vi "RT Host - normalised time profile.vi"(7 "Which speed profile?":T1, 8 "Error In":errorcluster, 11 "X Input (normalised 0-1)":dbl) -> (0 "Error Out":errorcluster, 2 "Profile Mean":dbl format="%0.2f", 3 "Y output (normalised 0-1)":dbl)   [LabVIEW 2017]
doc: "This subVI provides a Y-value according to a defined x-input by interpolating a senables multiple normailsed profiles to be created and followed according to."
uses:
  Controls/hCAAR - speed profile.ctl
  <vilib>/Analysis/baseanly.llb/Mean (DBL).vi
  <vilib>/Analysis/1siggen.llb/Ramp Pattern by Samples.vi
  <vilib>/Analysis/NI_AALPro.lvlib
  <vilib>/Analysis/NI_AALBase.lvlib
panel:
  out "Time V Distance Profile":cluster{dbl[], "Interpolant":dbl[]}(graph)={[0.0, 0.010101010101010102, 0.020202020202020204, 0.030303030303030304, 0.04040404040404041, 0.050505050505050504, 0.06060606060606061, 0.0707070707070707, 0.08080808080808081, 0.09090909090909091, 0.10101010101010101, 0.1111111111111111, 0.12121212121212122, 0.13131313131313133, 0.1414141414141414, 0.15151515151515152, 0.16161616161616163, 0.1717171717171717, 0.18181818181818182, 0.1919191919191919, 0.20202020202020202, 0.21212121212121213, 0.2222222222222222, 0.23232323232323232, 0.24242424242424243, 0.25252525252525254, 0.26262626262626265, 0.2727272727272727, 0.2828282828282828, 0.29292929292929293, 0.30303030303030304, 0.31313131313131315, 0.32323232323232326, 0.3333333333333333, 0.3434343434343434, 0.35353535353535354, 0.36363636363636365, 0.37373737373737376, 0.3838383838383838, 0.3939393939393939, 0.40404040404040403, 0.41414141414141414, 0.42424242424242425, 0.43434343434343436, 0.4444444444444444, 0.45454545454545453, 0.46464646464646464, 0.47474747474747475, 0.48484848484848486, 0.494949494949495, 0.5050505050505051, 0.5151515151515151, 0.5252525252525253, 0.5353535353535354, 0.5454545454545454, 0.5555555555555556, 0.5656565656565656, 0.5757575757575758, 0.5858585858585859, 0.5959595959595959, 0.6060606060606061, 0.6161616161616161, 0.6262626262626263, 0.6363636363636364, 0.6464646464646465, 0.6565656565656566, 0.6666666666666666, 0.6767676767676768, 0.6868686868686869, 0.696969696969697, 0.7070707070707071, 0.7171717171717171, 0.7272727272727273, 0.7373737373737373, 0.7474747474747475, 0.7575757575757576, 0.7676767676767676, 0.7777777777777778, 0.7878787878787878, 0.797979797979798, 0.8080808080808081, 0.8181818181818182, 0.8282828282828283, 0.8383838383838383, 0.8484848484848485, 0.8585858585858586, 0.8686868686868687, 0.8787878787878788, 0.8888888888888888, 0.898989898989899, 0.9090909090909091, 0.9191919191919192, 0.9292929292929293, 0.9393939393939394, 0.9494949494949495, 0.9595959595959596, 0.9696969696969697, 0.9797979797979798, 0.98989898989899, 1.0], "Interpolant"=[0.0, 0.03141075907812829, 0.06279051952931337, 0.09410831331851431, 0.12533323356430423, 0.15643446504023087, 0.1873813145857246, 0.21814324139654254, 0.24868988716485477, 0.2789911060392292, 0.3090169943749474, 0.33873792024529137, 0.3681245526846779, 0.3971478906347806, 0.4257792915650726, 0.4539904997395468, 0.4817536741017152, 0.5090414157503713, 0.5358267949789965, 0.5620833778521306, 0.587785252292473, 0.6129070536529765, 0.6374239897486896, 0.6613118653236518, 0.6845471059286886, 0.7071067811865475, 0.7289686274214114, 0.7501110696304595, 0.7705132427757891, 0.7901550123756903, 0.8090169943749473, 0.8270805742745617, 0.844327925502015, 0.8607420270039435, 0.8763066800438635, 0.8910065241883678, 0.9048270524660195, 0.917754625683981, 0.9297764858882513, 0.9408807689542253, 0.9510565162951535, 0.960293685676943, 0.9685831611286311, 0.9759167619387473, 0.9822872507286886, 0.9876883405951377, 0.9921147013144778, 0.99556196460308, 0.9980267284282716, 0.9995065603657316, 1.0, 0.9995065603657316, 0.9980267284282716, 0.9955619646030801, 0.9921147013144779, 0.9876883405951379, 0.9822872507286887, 0.9759167619387475, 0.9685831611286312, 0.9602936856769432, 0.9510565162951536, 0.9408807689542256, 0.9297764858882515, 0.9177546256839813, 0.9048270524660196, 0.891006524188368, 0.8763066800438637, 0.8607420270039438, 0.8443279255020152, 0.8270805742745619, 0.8090169943749476, 0.7901550123756905, 0.7705132427757894, 0.7501110696304597, 0.7289686274214117, 0.7071067811865477, 0.6845471059286888, 0.661311865323652, 0.6374239897486899, 0.6129070536529767, 0.5877852522924732, 0.5620833778521308, 0.5358267949789968, 0.5090414157503715, 0.48175367410171543, 0.453990499739547, 0.4257792915650728, 0.39714789063478084, 0.36812455268467814, 0.3387379202452916, 0.3090169943749476, 0.27899110603922944, 0.248689887164855, 0.21814324139654273, 0.18738131458572485, 0.15643446504023106, 0.12533323356430448, 0.09410831331851452, 0.06279051952931362, 0.03141075907812849]}
  out "Speed V Time Profile":cluster{dbl[], "Interpolant":dbl[]}(graph)={[0.0, 0.010101010101010102, 0.020202020202020204, 0.030303030303030304, 0.04040404040404041, 0.050505050505050504, 0.06060606060606061, 0.0707070707070707, 0.08080808080808081, 0.09090909090909091, 0.10101010101010101, 0.1111111111111111, 0.12121212121212122, 0.13131313131313133, 0.1414141414141414, 0.15151515151515152, 0.16161616161616163, 0.1717171717171717, 0.18181818181818182, 0.1919191919191919, 0.20202020202020202, 0.21212121212121213, 0.2222222222222222, 0.23232323232323232, 0.24242424242424243, 0.25252525252525254, 0.26262626262626265, 0.2727272727272727, 0.2828282828282828, 0.29292929292929293, 0.30303030303030304, 0.31313131313131315, 0.32323232323232326, 0.3333333333333333, 0.3434343434343434, 0.35353535353535354, 0.36363636363636365, 0.37373737373737376, 0.3838383838383838, 0.3939393939393939, 0.40404040404040403, 0.41414141414141414, 0.42424242424242425, 0.43434343434343436, 0.4444444444444444, 0.45454545454545453, 0.46464646464646464, 0.47474747474747475, 0.48484848484848486, 0.494949494949495, 0.5050505050505051, 0.5151515151515151, 0.5252525252525253, 0.5353535353535354, 0.5454545454545454, 0.5555555555555556, 0.5656565656565656, 0.5757575757575758, 0.5858585858585859, 0.5959595959595959, 0.6060606060606061, 0.6161616161616161, 0.6262626262626263, 0.6363636363636364, 0.6464646464646465, 0.6565656565656566, 0.6666666666666666, 0.6767676767676768, 0.6868686868686869, 0.696969696969697, 0.7070707070707071, 0.7171717171717171, 0.7272727272727273, 0.7373737373737373, 0.7474747474747475, 0.7575757575757576, 0.7676767676767676, 0.7777777777777778, 0.7878787878787878, 0.797979797979798, 0.8080808080808081, 0.8181818181818182, 0.8282828282828283, 0.8383838383838383, 0.8484848484848485, 0.8585858585858586, 0.8686868686868687, 0.8787878787878788, 0.8888888888888888, 0.898989898989899, 0.9090909090909091, 0.9191919191919192, 0.9292929292929293, 0.9393939393939394, 0.9494949494949495, 0.9595959595959596, 0.9696969696969697, 0.9797979797979798, 0.98989898989899, 1.0], "Interpolant"=[0.0, 0.03141075907812829, 0.06279051952931337, 0.09410831331851431, 0.12533323356430423, 0.15643446504023087, 0.1873813145857246, 0.21814324139654254, 0.24868988716485477, 0.2789911060392292, 0.3090169943749474, 0.33873792024529137, 0.3681245526846779, 0.3971478906347806, 0.4257792915650726, 0.4539904997395468, 0.4817536741017152, 0.5090414157503713, 0.5358267949789965, 0.5620833778521306, 0.587785252292473, 0.6129070536529765, 0.6374239897486896, 0.6613118653236518, 0.6845471059286886, 0.7071067811865475, 0.7289686274214114, 0.7501110696304595, 0.7705132427757891, 0.7901550123756903, 0.8090169943749473, 0.8270805742745617, 0.844327925502015, 0.8607420270039435, 0.8763066800438635, 0.8910065241883678, 0.9048270524660195, 0.917754625683981, 0.9297764858882513, 0.9408807689542253, 0.9510565162951535, 0.960293685676943, 0.9685831611286311, 0.9759167619387473, 0.9822872507286886, 0.9876883405951377, 0.9921147013144778, 0.99556196460308, 0.9980267284282716, 0.9995065603657316, 1.0, 0.9995065603657316, 0.9980267284282716, 0.9955619646030801, 0.9921147013144779, 0.9876883405951379, 0.9822872507286887, 0.9759167619387475, 0.9685831611286312, 0.9602936856769432, 0.9510565162951536, 0.9408807689542256, 0.9297764858882515, 0.9177546256839813, 0.9048270524660196, 0.891006524188368, 0.8763066800438637, 0.8607420270039438, 0.8443279255020152, 0.8270805742745619, 0.8090169943749476, 0.7901550123756905, 0.7705132427757894, 0.7501110696304597, 0.7289686274214117, 0.7071067811865477, 0.6845471059286888, 0.661311865323652, 0.6374239897486899, 0.6129070536529767, 0.5877852522924732, 0.5620833778521308, 0.5358267949789968, 0.5090414157503715, 0.48175367410171543, 0.453990499739547, 0.4257792915650728, 0.39714789063478084, 0.36812455268467814, 0.3387379202452916, 0.3090169943749476, 0.27899110603922944, 0.248689887164855, 0.21814324139654273, 0.18738131458572485, 0.15643446504023106, 0.12533323356430448, 0.09410831331851452, 0.06279051952931362, 0.03141075907812849]}
  in  "User-Defined":cluster{"X":dbl, "Y":dbl}[](array[cluster])=[{"X"=0.0, "Y"=0.0}, {"X"=0.0600000000000001, "Y"=0.13000000000000006}, {"X"=0.10999999999999996, "Y"=0.2999999999999998}, {"X"=0.17999999999999988, "Y"=0.5299999999999998}, {"X"=0.33999999999999997, "Y"=0.8599999999999999}, {"X"=0.47, "Y"=0.98}, {"X"=0.61, "Y"=0.99}, {"X"=0.8, "Y"=0.8600000000000001}, {"X"=0.8800000000000001, "Y"=0.5800000000000001}, {"X"=0.9500000000000001, "Y"=0.19000000000000006}, {"X"=1.0, "Y"=0.0}] {"Y" step=0.01; "X" step=0.01}
  # "Outputs"
  # "Inputs"
  # "Local Data"
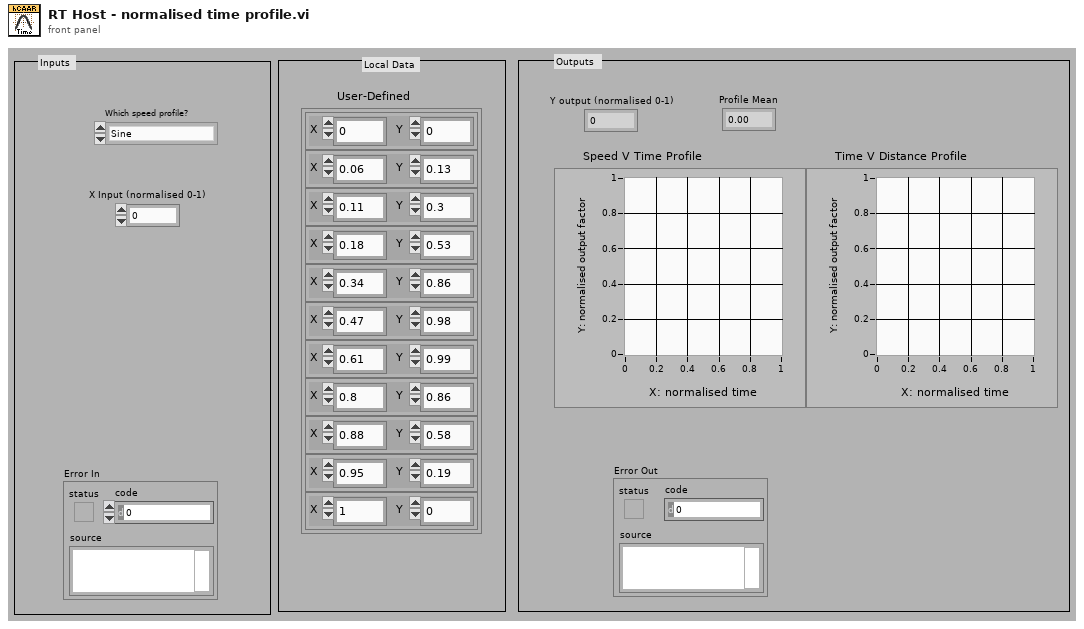
[diagram p1: front panel]
types:
  T1 = typedef "hCAAR - speed profile.ctl" = enum16{"Sine", "Sine With Initial Shunt", "Triangle", "Square", "Sawtooth", "Forward Skew", "User Defined"}
  T2 = enum16{"sine", "cosine", "triangle", "square", "sawtooth", "increasing ramp", "decreasing ramp"}
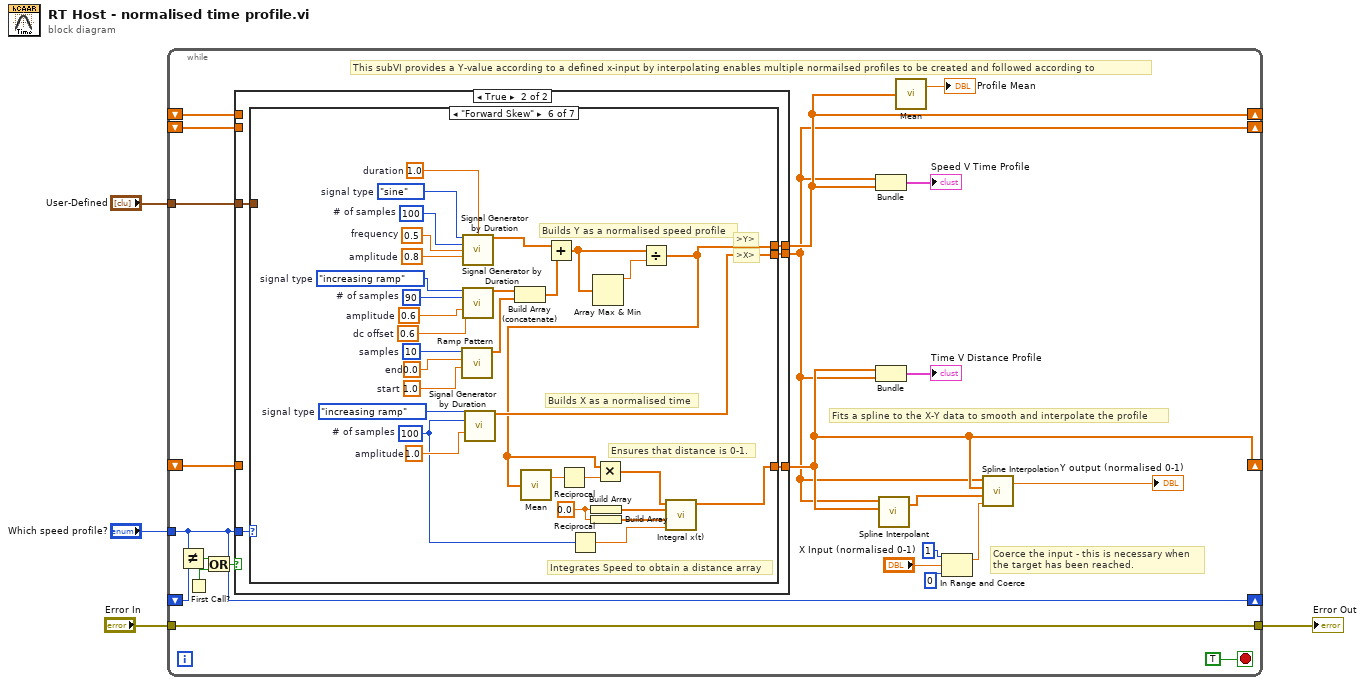
[diagram p0: block diagram]
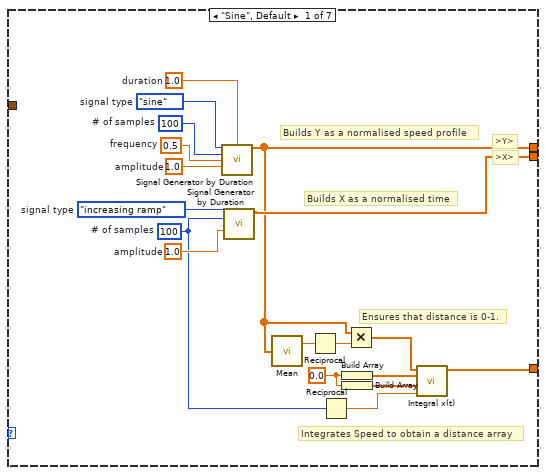
[diagram p3: hidden frame]
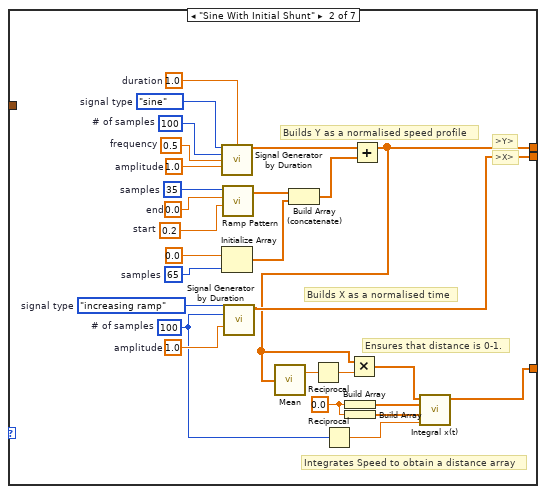
[diagram p4: hidden frame]
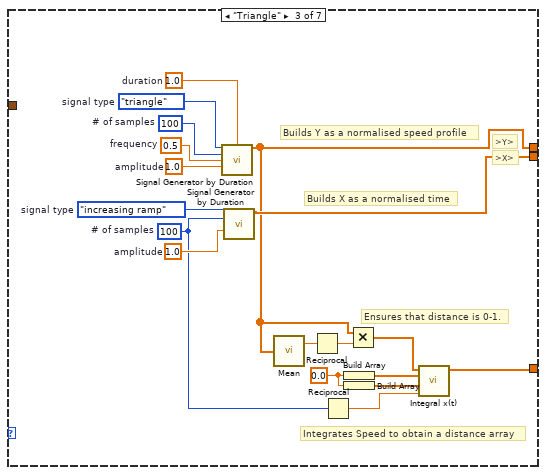
[diagram p5: hidden frame]
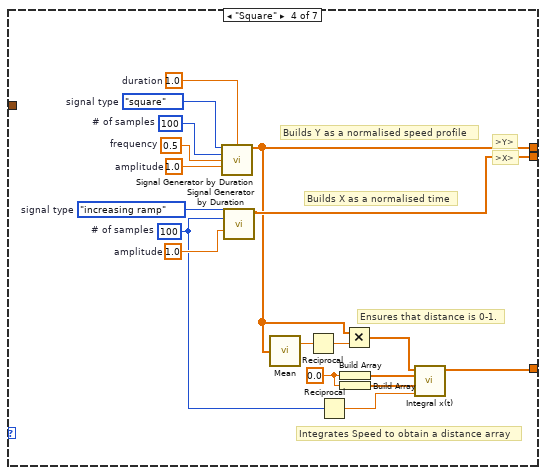
[diagram p6: hidden frame]
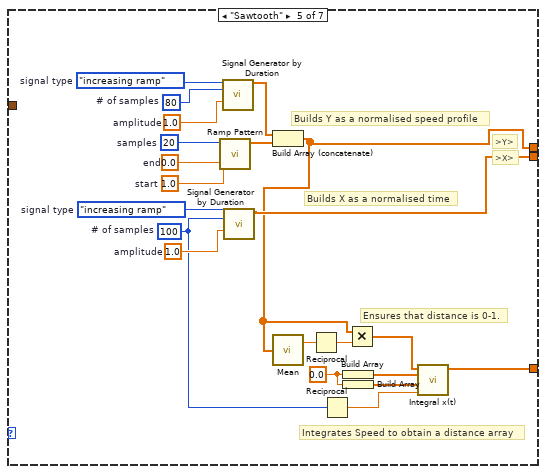
[diagram p7: hidden frame]
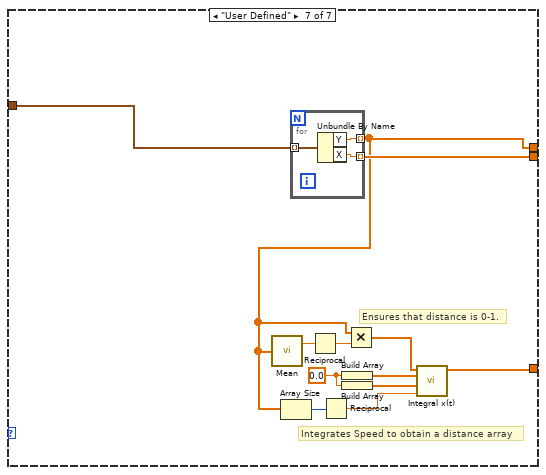
[diagram p8: hidden frame]
diagram:
  n1 = while {
    tunnel: "User-Defined" -> [w27]
    tunnel: "Which speed profile?" -> [w16]
    tunnel: [w20] -> w2
    tunnel: "Error In" -> [w20]
    shift-right: [w14] -> _
    shift-left: _ -> [w18]
    shift-right: [w6] -> _
    shift-left: _ -> [w17]
    shift-right: [w16] -> _
    shift-left: _ -> [w15]
    shift-right: [w7] -> _
    shift-left: _ -> [w9]
    stop <- TRUE stop-if-true
    # "This subVI provides a Y-value according to a defined x-input by interpolating enables multiple normailsed profiles to be created and followed according to"
    # "Fits a spline to the X-Y data to smooth and interpolate the profile"
    # "Coerce the input - this is necessary when\nthe target has been reached."
    n2 = Not Equal?(x=w16, y=w15) -> (x != y?=w12:bool)
    n3 = First Call?() -> (First Call?: T/F=w10:bool)
    n4 = Or(x=w12, y=w10) -> (x .or. y?=w11:bool)
    n5 = case shown="True" w11 {
      tunnel: w27 -> [_ w35]
      tunnel: w16 -> [_ w34]
      tunnel: [w29 w33] -> w6
      tunnel: [w30 w32] -> w14
      tunnel: w18 -> [w30 _]
      tunnel: w17 -> [w29 _]
      tunnel: [w28 w31] -> w7
      tunnel: w9 -> [w28 _]
      frame False {
        # "Saves CPU by only generating a new profile array when the profile type is changed"
      }
      frame True {
        n6 = case shown="\"Forward Skew\"" w34 {
          tunnel: [w46 w72 w91 w109 w135 w161 w180] -> w33
          tunnel: [w37 w55 w81 w100 w118 w139 w170] -> w32
          tunnel: w35 -> [_ _ _ _ _ _ w179]
          tunnel: [w38 w56 w86 w101 w119 w140 w171] -> w31
          frame "Sine", Default {
            w43 = 0.0
            w36 = 100  # # of samples
            w47 = 1.0  # amplitude
            w48 = T2."increasing ramp"  # signal type
            w49 = 1.0  # duration
            w50 = 100  # # of samples
            w51 = 0.5  # frequency
            w52 = 1.0  # amplitude
            w53 = T2."sine"  # signal type
            # "Ensures that distance is 0-1."
            # "Integrates Speed to obtain a distance array"
            # "Builds Y as a normalised speed profile"
            # "Builds X as a normalised time"
            # ">X>"
            # ">Y>"
            n7 = call <vilib>:"Signal Generator by Duration.vi"("signal type"=w53, "duration"=w49, "# of samples"=w50, "frequency"=w51, "amplitude"=w52) -> ("signal"=w37:dbl[])  [unwired: 7 in, 3 out]
            n8 = call <vilib>:"Signal Generator by Duration.vi"("signal type"=w48, "# of samples"=w36, "amplitude"=w47) -> ("signal"=w46:dbl[])  [unwired: 9 in, 3 out]
            n9 = call-poly <vilib>:"Mean.vi"("X"=w37) -> ("mean"=w41:dbl)  [unwired: 1 out]
            n10 = Reciprocal(x=w41) -> (1/x=w39:dbl)
            n11 = Reciprocal(x=w36) -> (1/x=w42:dbl)
            n12 = Build Array(w43) -> (w45:dbl[])
            n13 = Build Array(w43) -> (w44:dbl[])
            n14 = Multiply(x=w37, y=w39) -> (x*y=w40:dbl[])
            n15 = call <vilib>:"Integral x(t).vi"("dt"=w42, "Final Condition"=w44, "Initial Condition"=w45, "X"=w40) -> ("Integral X"=w38:dbl[])  [unwired: 6 in, 1 out]
          }
          frame "Sine With Initial Shunt" {
            w61 = 0.0
            w70 = 65  # samples
            w65 = 0.2  # start
            w67 = 0.0  # end
            w66 = 35  # samples
            w54 = 100  # # of samples
            w73 = 1.0  # amplitude
            w74 = T2."increasing ramp"  # signal type
            w76 = 1.0  # duration
            w77 = 100  # # of samples
            w78 = 0.5  # frequency
            w79 = 1.0  # amplitude
            w80 = T2."sine"  # signal type
            # "Ensures that distance is 0-1."
            # "Integrates Speed to obtain a distance array"
            # "Builds Y as a normalised speed profile"
            # "Builds X as a normalised time"
            # ">X>"
            # ">Y>"
            n16 = call <vilib>:"Signal Generator by Duration.vi"("signal type"=w80, "duration"=w76, "# of samples"=w77, "frequency"=w78, "amplitude"=w79) -> ("signal"=w75:dbl[])  [unwired: 7 in, 3 out]
            n17 = Initialize Array(0.0 ("element"), w70) -> (w71:dbl[])
            n18 = call-poly <vilib>:"Ramp Pattern.vi"("start"=w65, "end"=w67, "samples"=w66) -> ("Ramp Pattern"=w68:dbl[])  [unwired: 7 in, 1 out]
            n19 = call <vilib>:"Signal Generator by Duration.vi"("signal type"=w74, "# of samples"=w54, "amplitude"=w73) -> ("signal"=w72:dbl[])  [unwired: 9 in, 3 out]
            n20 = Build Array (concatenate)(w68, w71) -> (w64:dbl[])
            n21 = Reciprocal(x=w54) -> (1/x=w60:dbl)
            n22 = Build Array(w61) -> (w63:dbl[])
            n23 = Build Array(w61) -> (w62:dbl[])
            n24 = Add(x=w75, y=w64) -> (x+y=w55:dbl[])
            n25 = call-poly <vilib>:"Mean.vi"("X"=w55) -> ("mean"=w59:dbl)  [unwired: 1 out]
            n26 = Reciprocal(x=w59) -> (1/x=w57:dbl)
            n27 = Multiply(x=w55, y=w57) -> (x*y=w58:dbl[])
            n28 = call <vilib>:"Integral x(t).vi"("dt"=w60, "Final Condition"=w62, "Initial Condition"=w63, "X"=w58) -> ("Integral X"=w56:dbl[])  [unwired: 6 in, 1 out]
          }
          frame "Triangle" {
            w88 = 0.0
            w85 = 100  # # of samples
            w92 = 1.0  # amplitude
            w93 = T2."increasing ramp"  # signal type
            w94 = 1.0  # duration
            w95 = 100  # # of samples
            w96 = 0.5  # frequency
            w97 = 1.0  # amplitude
            w98 = T2."triangle"  # signal type
            # "Ensures that distance is 0-1."
            # "Integrates Speed to obtain a distance array"
            # "Builds Y as a normalised speed profile"
            # "Builds X as a normalised time"
            # ">X>"
            # ">Y>"
            n29 = call <vilib>:"Signal Generator by Duration.vi"("signal type"=w98, "duration"=w94, "# of samples"=w95, "frequency"=w96, "amplitude"=w97) -> ("signal"=w81:dbl[])  [unwired: 7 in, 3 out]
            n30 = call <vilib>:"Signal Generator by Duration.vi"("signal type"=w93, "# of samples"=w85, "amplitude"=w92) -> ("signal"=w91:dbl[])  [unwired: 9 in, 3 out]
            n31 = call-poly <vilib>:"Mean.vi"("X"=w81) -> ("mean"=w84:dbl)  [unwired: 1 out]
            n32 = Reciprocal(x=w84) -> (1/x=w82:dbl)
            n33 = Reciprocal(x=w85) -> (1/x=w87:dbl)
            n34 = Build Array(w88) -> (w90:dbl[])
            n35 = Build Array(w88) -> (w89:dbl[])
            n36 = Multiply(x=w81, y=w82) -> (x*y=w83:dbl[])
            n37 = call <vilib>:"Integral x(t).vi"("dt"=w87, "Final Condition"=w89, "Initial Condition"=w90, "X"=w83) -> ("Integral X"=w86:dbl[])  [unwired: 6 in, 1 out]
          }
          frame "Square" {
            w106 = 0.0
            w99 = 100  # # of samples
            w110 = 1.0  # amplitude
            w111 = T2."increasing ramp"  # signal type
            w112 = 1.0  # duration
            w113 = 100  # # of samples
            w114 = 0.5  # frequency
            w115 = 1.0  # amplitude
            w116 = T2."square"  # signal type
            # "Ensures that distance is 0-1."
            # "Integrates Speed to obtain a distance array"
            # "Builds Y as a normalised speed profile"
            # "Builds X as a normalised time"
            # ">X>"
            # ">Y>"
            n38 = call <vilib>:"Signal Generator by Duration.vi"("signal type"=w116, "duration"=w112, "# of samples"=w113, "frequency"=w114, "amplitude"=w115) -> ("signal"=w100:dbl[])  [unwired: 7 in, 3 out]
            n39 = call <vilib>:"Signal Generator by Duration.vi"("signal type"=w111, "# of samples"=w99, "amplitude"=w110) -> ("signal"=w109:dbl[])  [unwired: 9 in, 3 out]
            n40 = call-poly <vilib>:"Mean.vi"("X"=w100) -> ("mean"=w104:dbl)  [unwired: 1 out]
            n41 = Reciprocal(x=w104) -> (1/x=w102:dbl)
            n42 = Reciprocal(x=w99) -> (1/x=w105:dbl)
            n43 = Build Array(w106) -> (w108:dbl[])
            n44 = Build Array(w106) -> (w107:dbl[])
            n45 = Multiply(x=w100, y=w102) -> (x*y=w103:dbl[])
            n46 = call <vilib>:"Integral x(t).vi"("dt"=w105, "Final Condition"=w107, "Initial Condition"=w108, "X"=w103) -> ("Integral X"=w101:dbl[])  [unwired: 6 in, 1 out]
          }
          frame "Sawtooth" {
            w124 = 0.0
            w127 = 1.0  # start
            w128 = 0.0  # end
            w129 = 20  # samples
            w133 = 80  # # of samples
            w134 = 1.0  # amplitude
            w132 = T2."increasing ramp"  # signal type
            w117 = 100  # # of samples
            w136 = 1.0  # amplitude
            w137 = T2."increasing ramp"  # signal type
            # "Ensures that distance is 0-1."
            # "Integrates Speed to obtain a distance array"
            # "Builds Y as a normalised speed profile"
            # "Builds X as a normalised time"
            # ">X>"
            # ">Y>"
            n47 = call-poly <vilib>:"Ramp Pattern.vi"("start"=w127, "end"=w128, "samples"=w129) -> ("Ramp Pattern"=w130:dbl[])  [unwired: 7 in, 1 out]
            n48 = call <vilib>:"Signal Generator by Duration.vi"("signal type"=w132, "# of samples"=w133, "amplitude"=w134) -> ("signal"=w131:dbl[])  [unwired: 9 in, 3 out]
            n49 = call <vilib>:"Signal Generator by Duration.vi"("signal type"=w137, "# of samples"=w117, "amplitude"=w136) -> ("signal"=w135:dbl[])  [unwired: 9 in, 3 out]
            n50 = Build Array (concatenate)(w131, w130) -> (w118:dbl[])
            n51 = call-poly <vilib>:"Mean.vi"("X"=w118) -> ("mean"=w122:dbl)  [unwired: 1 out]
            n52 = Reciprocal(x=w122) -> (1/x=w120:dbl)
            n53 = Reciprocal(x=w117) -> (1/x=w123:dbl)
            n54 = Build Array(w124) -> (w126:dbl[])
            n55 = Build Array(w124) -> (w125:dbl[])
            n56 = Multiply(x=w118, y=w120) -> (x*y=w121:dbl[])
            n57 = call <vilib>:"Integral x(t).vi"("dt"=w123, "Final Condition"=w125, "Initial Condition"=w126, "X"=w121) -> ("Integral X"=w119:dbl[])  [unwired: 6 in, 1 out]
          }
          frame "Forward Skew" {
            w145 = 0.0
            w148 = 0.6  # dc offset
            w152 = 1.0  # start
            w154 = 0.0  # end
            w153 = 10  # samples
            w159 = 90  # # of samples
            w160 = 0.6  # amplitude
            w158 = T2."increasing ramp"  # signal type
            w138 = 100  # # of samples
            w162 = 1.0  # amplitude
            w163 = T2."increasing ramp"  # signal type
            w164 = 1.0  # duration
            w165 = 100  # # of samples
            w166 = 0.5  # frequency
            w167 = 0.8  # amplitude
            w168 = T2."sine"  # signal type
            # "Ensures that distance is 0-1."
            # "Integrates Speed to obtain a distance array"
            # "Builds Y as a normalised speed profile"
            # "Builds X as a normalised time"
            # ">X>"
            # ">Y>"
            n58 = call-poly <vilib>:"Ramp Pattern.vi"("start"=w152, "end"=w154, "samples"=w153) -> ("Ramp Pattern"=w151:dbl[])  [unwired: 7 in, 1 out]
            n59 = call <vilib>:"Signal Generator by Duration.vi"("signal type"=w168, "duration"=w164, "# of samples"=w165, "frequency"=w166, "amplitude"=w167) -> ("signal"=w157:dbl[])  [unwired: 7 in, 3 out]
            n60 = call <vilib>:"Signal Generator by Duration.vi"("signal type"=w158, "# of samples"=w159, "amplitude"=w160, "dc offset"=w148) -> ("signal"=w156:dbl[])  [unwired: 8 in, 3 out]
            n61 = call <vilib>:"Signal Generator by Duration.vi"("signal type"=w163, "# of samples"=w138, "amplitude"=w162) -> ("signal"=w161:dbl[])  [unwired: 9 in, 3 out]
            n62 = Build Array (concatenate)(w156, w151) -> (w155:dbl[])
            n63 = Add(x=w157, y=w155) -> (x+y=w149:dbl[])
            n64 = Reciprocal(x=w138) -> (1/x=w144:dbl)
            n65 = Build Array(w145) -> (w147:dbl[])
            n66 = Build Array(w145) -> (w146:dbl[])
            n67 = Array Max & Min(array=w149) -> (max value=w150:dbl)  [unwired: 3 out]
            n68 = Divide(x=w149, y=w150) -> (x/y=w139:dbl[])
            n69 = call-poly <vilib>:"Mean.vi"("X"=w139) -> ("mean"=w143:dbl)  [unwired: 1 out]
            n70 = Reciprocal(x=w143) -> (1/x=w141:dbl)
            n71 = Multiply(x=w139, y=w141) -> (x*y=w142:dbl[])
            n72 = call <vilib>:"Integral x(t).vi"("dt"=w144, "Final Condition"=w146, "Initial Condition"=w147, "X"=w142) -> ("Integral X"=w140:dbl[])  [unwired: 6 in, 1 out]
          }
          frame "User Defined" {
            w176 = 0.0
            # "Ensures that distance is 0-1."
            # "Integrates Speed to obtain a distance array"
            n73 = for {
              tunnel: w179 -> [w183] mode=indexing
              tunnel: [w182] -> w170 mode=indexing
              tunnel: [w181] -> w180 mode=indexing
              n74 = Unbundle By Name(w183) -> ("Y"=w182:dbl, "X"=w181:dbl)
            }
            n75 = call-poly <vilib>:"Mean.vi"("X"=w170) -> ("mean"=w174:dbl)  [unwired: 1 out]
            n76 = Array Size(array=w170) -> (size(s)=w169:i32)
            n77 = Reciprocal(x=w174) -> (1/x=w172:dbl)
            n78 = Reciprocal(x=w169) -> (1/x=w175:dbl)
            n79 = Build Array(w176) -> (w178:dbl[])
            n80 = Build Array(w176) -> (w177:dbl[])
            n81 = Multiply(x=w170, y=w172) -> (x*y=w173:dbl[])
            n82 = call <vilib>:"Integral x(t).vi"("dt"=w175, "Final Condition"=w177, "Initial Condition"=w178, "X"=w173) -> ("Integral X"=w171:dbl[])  [unwired: 6 in, 1 out]
          }
        }
      }
    }
    n83 = Bundle("signal"=w6, "signal"=w14) -> (→"Speed V Time Profile":cluster{"signal":dbl[], "signal":dbl[]})  [unwired: 1 in]
    n84 = Bundle("Integral X"=w7, "signal"=w6) -> (→"Time V Distance Profile":cluster{"Integral X":dbl[], "signal":dbl[]})  [unwired: 1 in]
    n85 = call <vilib>:"Spline Interpolant.vi"("X"=w7, "Y"=w6) -> ("Interpolant"=w22:dbl[])  [unwired: 2 in, 1 out]
    n86 = call-poly <vilib>:"Mean.vi"("X"=w14) -> ("mean"=→"Profile Mean":dbl)  [unwired: 1 out]
    n87 = In Range and Coerce(upper limit=1, x="X Input (normalised 0-1)", lower limit=0) -> (coerced(x)=w25:dbl)  [unwired: 1 out]
    n88 = call <vilib>:"Spline Interpolation.vi"("x value"=w25, "Interpolant"=w22, "X"=w7, "Y"=w6) -> ("interpolation value"=→"Y output (normalised 0-1)":dbl)  [unwired: 1 out]
  }
  "Error Out" <- w2
